vi "Cal Data save to DB.vi"(8 "Error In":errorcluster, 9 "Model (F-ME74)":bool, 10 "Adjusted Amplitude":dbl[](array[numeric]), 11 "DB File":path) -> (0 "Error Out":errorcluster)   [LabVIEW 2018]
uses:
  <vilib>/drjdpowell/SQLite Library/SQL Connection/Connection.lvclass/Connection.ctl
  <vilib>/drjdpowell/SQLite Library/SQL Connection/Open (path).vi
  <vilib>/drjdpowell/SQLite Library/SQL Connection/Open (string).vi
  <vilib>/AdvancedString/Path To Command Line String.vi
  <vilib>/drjdpowell/SQLite Library/SQL Connection/Execute SQL (No results).vi
  <vilib>/drjdpowell/SQLite Library/SQL Connection/Connection.lvclass
  <vilib>/drjdpowell/SQLite Library/SQLite.lvlib
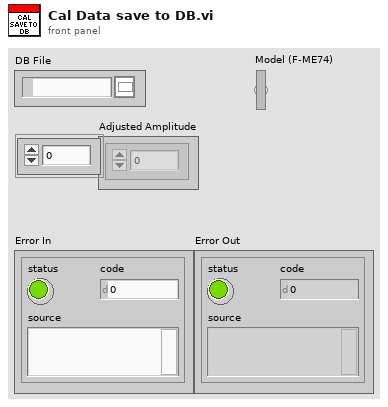
[diagram p1: front panel]
types:
  T1 = enum16{"New or existing", "Existing", "Read only"}
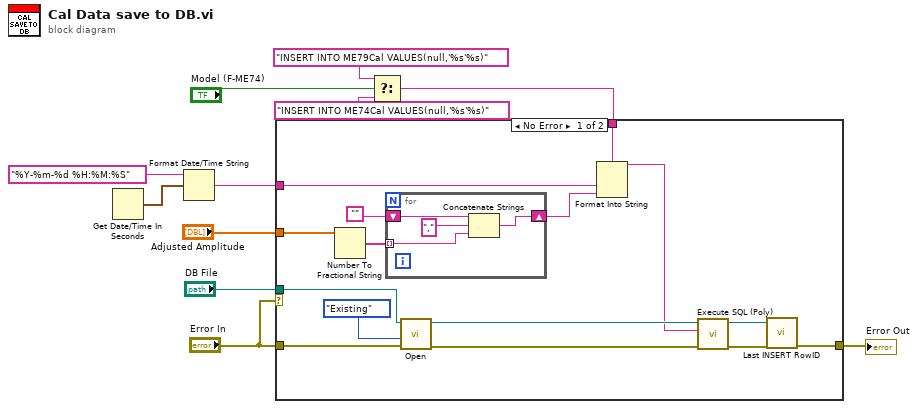
[diagram p0: block diagram]
diagram:
  n1 = Get Date/Time In Seconds() -> (seconds since 1Jan1904=w9:timestamp)
  n2 = Format Date/Time String(time format string (%c)="%Y-%m-%d %H:%M:%S", seconds (now)=w9) -> (date/time string=w7:string)  [unwired: 1 in]
  n3 = Select(t="INSERT INTO ME79Cal VALUES(null,'%s'%s)", s="Model (F-ME74)", f="INSERT INTO ME74Cal VALUES(null,'%s'%s)") -> (s? t:f=w1:string)
  n4 = case shown="No Error" "Error In" {
    tunnel: "Error In" -> [w25 w31]
    tunnel: "DB File" -> [w24 _]
    tunnel: w7 -> [w22 _]
    tunnel: "Adjusted Amplitude" -> [w21 _]
    tunnel: [w13 w31] -> w5
    tunnel: w1 -> [w12 _]
    frame No Error {
      n5 = Number To Fractional String(number=w21) -> (F-format string=w20:string[])  [unwired: 3 in]
      n6 = for {
        tunnel: w20 -> [w28] mode=indexing
        shift-right: [w27] -> w18
        shift-left: "" -> [w30]
        n7 = Concatenate Strings(w30, ",", w28) -> (w27:string)
      }
      n8 = call-poly <vilib>:"Open.vi"("error in (no error)"=w25, "File Option"=T1."Existing", "db file"=w24) -> ("error out"=w23:errorcluster, "SQLite Connection"=w17:refnum<class "Connection.lvclass">)  [unwired: 7 in]
      n9 = Format Into String(format string=w12, w22, w18) -> (resulting string=w16:string)  [unwired: 2 in, 1 out]
      n10 = call-poly <vilib>:"Execute SQL (Poly).vi"("error in (no error)"=w23, "SQL"=w16, "SQLite Connection in"=w17) -> ("error out"=w15:errorcluster, "SQLite Connection"=w14:refnum<class "Connection.lvclass">)  [unwired: 7 in]
      n11 = call <vilib>:"Last INSERT RowID.vi"("error in (no error)"=w15, "SQLite Connection in"=w14) -> ("error out"=w13:errorcluster)  [unwired: 7 in, 2 out]
    }
    frame Error {
    }
  }
  "Error Out" <- w5
